vi "UsingParameterisedQuery.vi"() -> ()   [LabVIEW 2019]
uses:
  <vilib>/addons/database/Auxilliary.llb/DB Tools Parameter Info.ctl
  <vilib>/addons/database/Auxilliary.llb/DB Tools DataTypes.ctl
  <vilib>/addons/database/Auxilliary.llb/DB Tools Parameter Dir.ctl
  <vilib>/addons/database/Connection.llb/DB Tools Open Connec (String).vi
  <vilib>/addons/database/Command.llb/Cmd Set Parameter Value (C).vi
  <vilib>/addons/database/Command.llb/Cmd Execute.vi
  <vilib>/addons/database/Recordset.llb/Rec Destroy - Command.vi
  <vilib>/addons/database/Command.llb/Cmd Delete.vi
  <vilib>/addons/database/NI_Database_API.lvlib
panel:
  in  "Salary":dbl
  in  "PassFail":bool
  in  "Marks":dbl
  in  "Serial No":dbl
  in  "Subject Name":string
  in  "stop":bool
  in  "Provide your ODBC server name":string
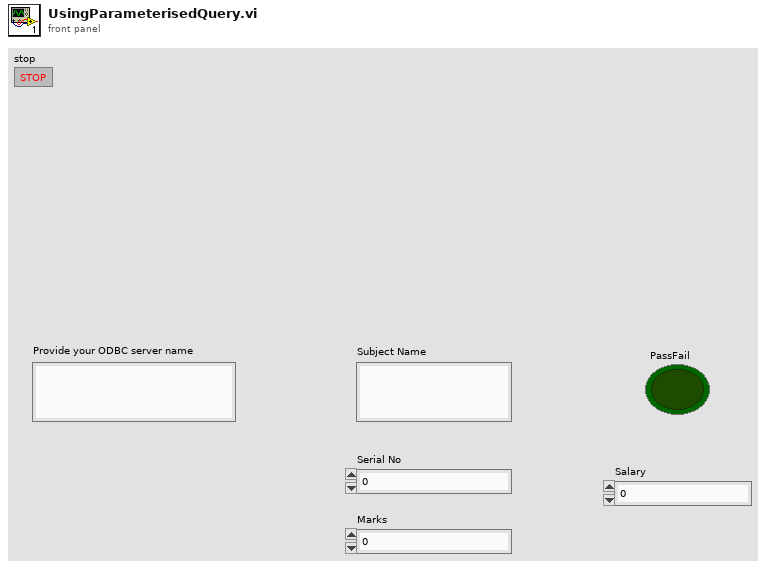
[diagram p1: front panel]
types:
  T1 = typedef "NI_Database_API.lvlib/DB Tools Parameter Info.ctl" = cluster{"parameter name":string, "type":T2, "direction":T3, "value":variant}
  T2 = typedef "NI_Database_API.lvlib/DB Tools DataTypes.ctl" = enum16{"String", "Long (I32)", "Single (SGL)", "Double (DBL)", "Date/Time", "Binary"}
  T3 = typedef "NI_Database_API.lvlib/DB Tools Parameter Dir.ctl" = enum32{"Input", "Output", "Input/Output", "Return Value"}
  T4 = typedef "NI_Database_API.lvlib/Conn ObjectReference.ctl" = refnum<k1>
  T5 = typedef "NI_Database_API.lvlib/Cmd ObjectReference.ctl" = refnum<k1>
  T6 = typedef "NI_Database_API.lvlib/Cmd-Rec Object Reference.ctl" = refnum<k1>
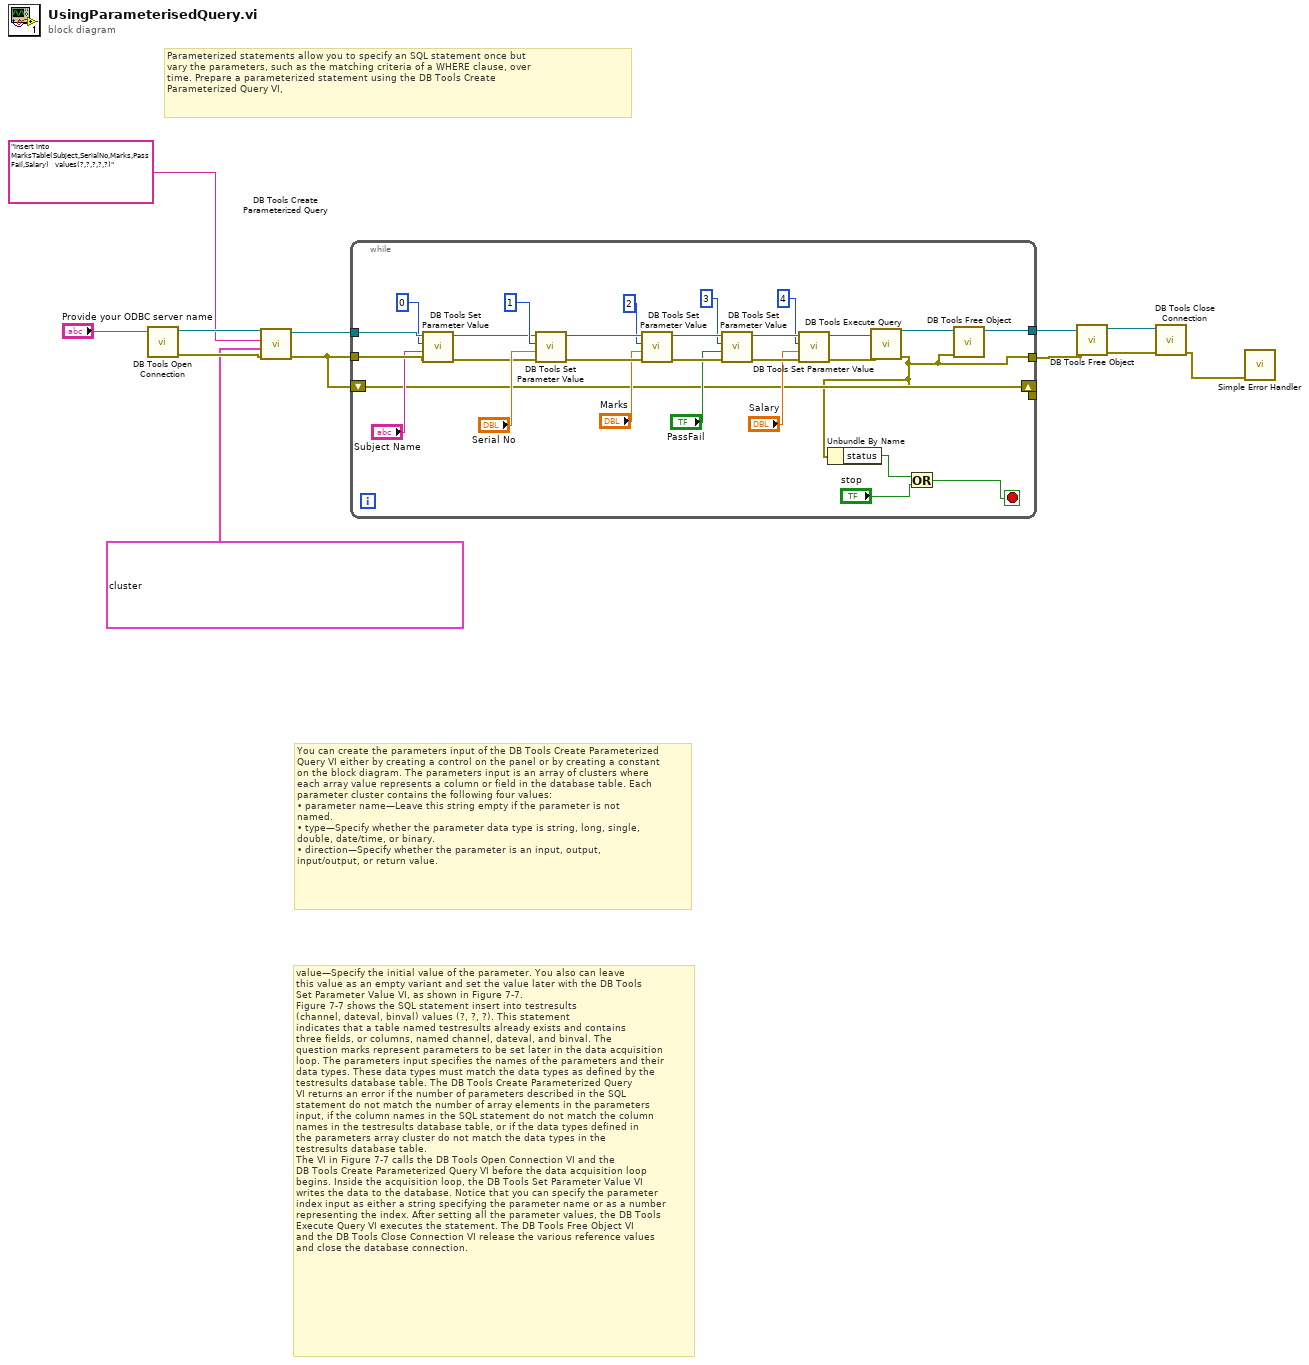
[diagram p0: block diagram]
diagram:
  # "value—Specify the initial value of the parameter. You also can leave\nthis value as an empty variant and set the value later with the DB Tools\nSet Parameter Value VI, as shown in Figure 7-7.\nFigure 7-7 shows the SQL statement insert into testresults\n(channel, dateval, binval) values (?, ?, ?). This statement\nindicates that a table named testresults already exists and contains\nthree fields, or columns, named channel, dateval, and binval. The\nquestion marks represent parameters to be set later in the data acquisition\nloop. The parameters input specifies the names of the parameters and their\ndata types. These data types must match the data types as defined by the\ntestresults database table. The DB Tools Create Parameterized Query\nVI returns an error if the number of parameters described in the SQL\nstatement do not match the number of array elements in the parameters\ninput, if the column names in the SQL statement do not match the column\nnames in the testresults database table, or if the data types defined in\nthe parameters array cluster do not match the data types in the\ntestresults database table.\nThe VI in Figure 7-7 calls the DB Tools Open Connection VI and the\nDB Tools Create Parameterized Query VI before the data acquisition loop\nbegins. Inside the acquisition loop, the DB Tools Set Parameter Value VI\nwrites the data to the database. Notice that you can specify the parameter\nindex input as either a string specifying the parameter name or as a number\nrepresenting the index. After setting all the parameter values, the DB Tools\nExecute Query VI executes the statement. The DB Tools Free Object VI\nand the DB Tools Close Connection VI release the various reference values\nand close the database connection."
  # "You can create the parameters input of the DB Tools Create Parameterized\nQuery VI either by creating a control on the panel or by creating a constant\non the block diagram. The parameters input is an array of clusters where\neach array value represents a column or field in the database table. Each\nparameter cluster contains the following four values:\n• parameter name—Leave this string empty if the parameter is not\nnamed.\n• type—Specify whether the parameter data type is string, long, single,\ndouble, date/time, or binary.\n• direction—Specify whether the parameter is an input, output,\ninput/output, or return value."
  # "Parameterized statements allow you to specify an SQL statement once but\nvary the parameters, such as the matching criteria of a WHERE clause, over\ntime. Prepare a parameterized statement using the DB Tools Create\nParameterized Query VI,"
  n1 = call-poly <vilib>:"DB Tools Open Connection.vi"("connection information"="Provide your ODBC server name") -> ("error out"=w10:errorcluster, "connection reference"=w11:T4)  [unwired: 7 in]
  n2 = call <vilib>:"DB Tools Create Parameterized Query.vi"("error in (no error)"=w10, "parameters"=T1[] [{"parameter name"="Subject", "type"=enum."String", "direction"=enum."Output", "value"=variant}, {"parameter name"="SerialNo", "type"=enum."Long (I32)", "direction"=enum."Output", "value"=variant}, {"parameter name"="Marks", "type"=enum."Double (DBL)", "direction"=enum."Output", "value"=variant}, {"parameter name"="PassFail", "type"=enum."Binary", "direction"=enum."Output", "value"=variant}, {"parameter name"="Salary", "type"=enum."Double (DBL)", "direction"=enum."Output", "value"=variant}], "SQL query"="insert into MarksTable(Subject,SerialNo,Marks,PassFail,Salary)   values(?,?,?,?,?)", "connection reference"=w11) -> ("error out"=w6:errorcluster, "command reference"=w7:T5)  [unwired: 3 in, 1 out]
  n3 = while {
    tunnel: w7 -> [w41]
    tunnel: w6 -> [w40]
    shift-right: [w16] -> _
    shift-left: w6 -> [w19]
    tunnel: [w19] -> _
    tunnel: [w16] -> w5
    tunnel: [w17] -> w2
    stop <- w13 stop-if-true
    n4 = call-poly <vilib>:"DB Tools Set Parameter Value.vi"("error in (no error)"=w40, "value"="Subject Name", "parameter index"=0, "command reference"=w41) -> ("error out"=w34:errorcluster, "command reference out"=w35:T5)  [unwired: 4 in]
    n5 = call-poly <vilib>:"DB Tools Set Parameter Value.vi"("error in (no error)"=w34, "value"="Serial No", "parameter index"=1, "command reference"=w35) -> ("error out"=w32:errorcluster, "command reference out"=w33:T5)  [unwired: 4 in]
    n6 = call-poly <vilib>:"DB Tools Set Parameter Value.vi"("error in (no error)"=w32, "value"="Marks", "parameter index"=2, "command reference"=w33) -> ("error out"=w28:errorcluster, "command reference out"=w29:T5)  [unwired: 4 in]
    n7 = call-poly <vilib>:"DB Tools Set Parameter Value.vi"("error in (no error)"=w28, "value"="PassFail", "parameter index"=3, "command reference"=w29) -> ("error out"=w24:errorcluster, "command reference out"=w25:T5)  [unwired: 4 in]
    n8 = call-poly <vilib>:"DB Tools Set Parameter Value.vi"("error in (no error)"=w24, "value"="Salary", "parameter index"=4, "command reference"=w25) -> ("error out"=w20:errorcluster, "command reference out"=w21:T5)  [unwired: 4 in]
    n9 = call-poly <vilib>:"DB Tools Execute Query.vi"("error in (no error)"=w20, "command reference"=w21) -> ("error out"=w16:errorcluster, "command-recordset reference"=w18:T6)  [unwired: 6 in]
    n10 = Unbundle By Name(w16) -> ("status"=w15:bool)
    n11 = Or(x=w15, y="stop") -> (x .or. y?=w13:bool)
    n12 = call-poly <vilib>:"DB Tools Free Object.vi"("error in (no error)"=w16, "command-recordset reference"=w18) -> ("command reference"=w17:T5)  [unwired: 8 in, 1 out]
  }
  n13 = call-poly <vilib>:"DB Tools Free Object.vi"("error in (no error)"=w5, "command reference"=w2) -> ("error out"=w4:errorcluster, "connection reference"=w3:T4)  [unwired: 8 in]
  n14 = call <vilib>:"DB Tools Close Connection.vi"("error in (no error)"=w4, "connection reference"=w3) -> ("error out"=w1:errorcluster)  [unwired: 5 in]
  n15 = call <vilib>:"Simple Error Handler.vi"("error in (no error)"=w1) -> ()  [unwired: 4 in, 5 out]
